vi "dfd_FXP PtByPt Odd Symmetric FIR.vi"(6 "state in":i64[](array[numeric]), 7 "FXPOPs":T5[](array[typedef]) {"source" items=["Coef a/k"=0, "Coef b/v"=7, "Input"=1, "Output"=2, "Multiplicand"=3, "Product"=4, "Sum"=5, "Delay"=6, "Gain"=8]}, 8 "filtering statistics in":T4(array[cluster]) {"statistics information"."min value" format="%.2f"; "statistics information"."max value" format="%.2f"; "Quantizer Source" items=["Coefficients a/k"=0, "Coefficients b/v"=7, "Input"=1, "Output"=2, "Multiplicand"=3, "Product"=4, "Sum"=5, "Delay"=6]}, 10 "coef b (half stored)":i64[](array[numeric]), 11 "x":T7={"value"=0, "wl"=0, "iwl"=0, "Signed"=TRUE} {"value" format="%.0x"}) -> (0 "filtering statistics out":T4(array[cluster]) {"statistics information"."min value" format="%.2f"; "statistics information"."max value" format="%.2f"; "Quantizer Source" items=["Coefficients a/k"=0, "Coefficients b/v"=7, "Input"=1, "Output"=2, "Multiplicand"=3, "Product"=4, "Sum"=5, "Delay"=6]}, 3 "filtered x":T7={"value"=0, "wl"=0, "iwl"=0, "Signed"=TRUE} {"value" format="%.0x"}, 4 "state out":i64[](array[numeric]))   [LabVIEW 2017, in "NI_DigFilter_FXP.lvlib"]
uses:
  <vilib>/addons/Digital Filter Design/NI_DigFilter_FXP.lvlib
  <vilib>/addons/Digital Filter Design/_Objects.llb/dfd_DFXP Data Type (scaler).ctl
  <vilib>/addons/Digital Filter Design/_Objects.llb/dfd_DFXP Operation Parameter.ctl
  <vilib>/addons/Digital Filter Design/_Objects.llb/dfd_Internal Quantization Srcs.ctl
  <vilib>/addons/Digital Filter Design/_Objects.llb/DFD Quantization Sources.ctl
  <vilib>/addons/Digital Filter Design/_Objects.llb/DFD FXP Statistics Data.ctl
  <vilib>/addons/Digital Filter Design/_Objects.llb/dfd_DFXP Data Type (vector).ctl
  <vilib>/addons/Digital Filter Design/NI_DigFilterLicensed.lvlib
panel:
  in  "DFXP type":T1
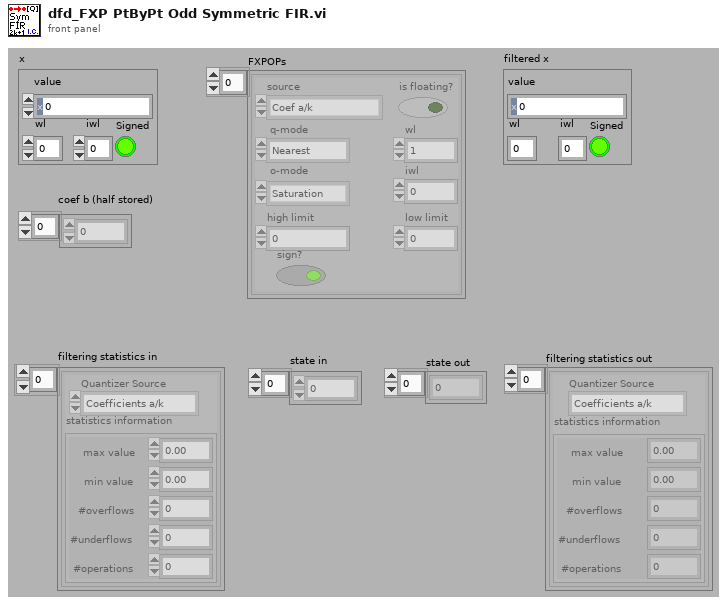
[diagram p1: front panel]
types:
  T1 = typedef "dfd_DFXP Data Type (vector).ctl" = cluster{"Values":i64[], "wl":i16, "iwl":i16}
  T2 = typedef "NI_DigFilterLicensed.lvlib/DFD Quantization Sources.ctl" = u16
  T3 = typedef "NI_DigFilterLicensed.lvlib/DFD FXP Statistics Data.ctl" = cluster{"max value":ext, "min value":ext, "#overflows":i32, "#underflows":i32, "#operations":i32}
  T4 = cluster{"Quantizer Source":T2, "statistics information":T3}[]
  T5 = typedef "dfd_DFXP Operation Parameter.ctl" = cluster{"source":T6, "is floating?":bool, "o-mode":enum16{"Saturation", "Wrap"}, "q-mode":enum16{"Nearest", "Truncation"}, "wl":i16, "high limit":i64, "low limit":i64, "iwl":i16, "sign?":bool}
  T6 = typedef "NI_DigFilterLicensed.lvlib/dfd_Internal Quantization Srcs.ctl" = u16
  T7 = typedef "dfd_DFXP Data Type (scaler).ctl" = cluster{"value":i64, "wl":i16, "iwl":i16, "Signed":bool}
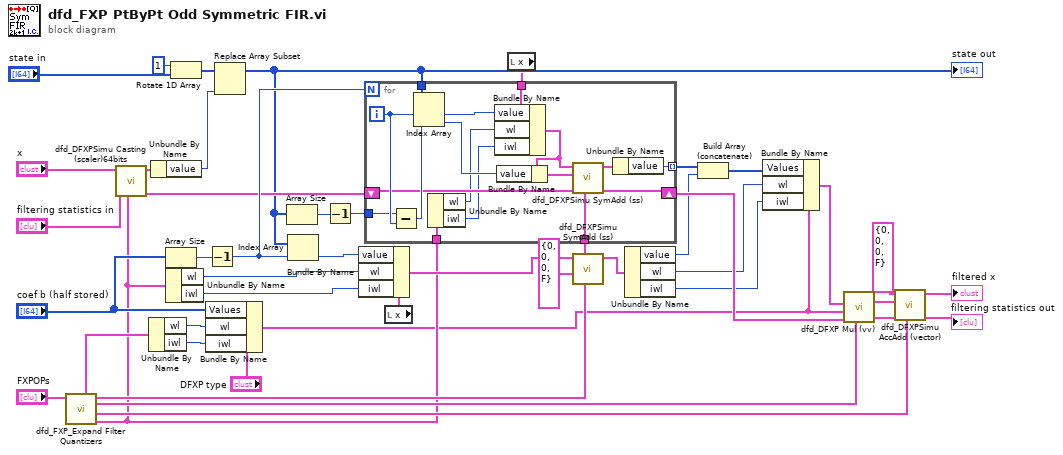
[diagram p0: block diagram]
diagram:
  n1 = call <vilib>:"dfd_FXP_Expand Filter Quantizers.vi"("FXPOPs"="FXPOPs") -> ("Delay"=w8:T5, "Sum"=w32:T5, "Product"=w33:T5, "Multiplicand"=w26:T5, "Coefficient b/v"=w16:T5)  [unwired: 6 out]
  n2 = call <vilib>:"dfd_DFXPSimu Casting (scaler)64bits.vi"("op params"=w8, "filtering statistics in"="filtering statistics in", "Value in"="x") -> ("filtering statistics out"=w29:T4, "Value out"=w20:T7)  [unwired: 1 in, 6 out]
  n3 = Unbundle By Name(w16) -> ("wl"=w13:i16, "iwl"=w12:i16)
  n4 = Unbundle By Name(w20) -> ("value"=w9:i64)
  n5 = Array Size(array="coef b (half stored)") -> (size(s)=w42:i32)
  n6 = Unbundle By Name(w8) -> ("wl"=w11:i16, "iwl"=w10:i16)
  n7 = Rotate 1D Array(1:"state in", 2:1 ("n")) -> (0:w44:i64[])
  n8 = Bundle By Name(cluster="DFXP type", "Values"="coef b (half stored)", "wl"=w13, "iwl"=w12) -> (w5:T1)
  n9 = Decrement(x=w42) -> (x-1=w31:i32)
  n10 = Replace Array Subset(array=w44, new element=w9) -> (w22:i64[])  [unwired: 1 in]
  "state out" <- w22
  n11 = Array Size(array=w22) -> (size(s)=w40:i32)
  n12 = Index Array(array=w22, index=w31) -> (element=w27:i64)
  n13 = Decrement(x=w40) -> (x-1=w38:i32)
  n14 = local read "x"() -> (w14:T7)
  n15 = Bundle By Name(cluster=w14, "value"=w27, "wl"=w11, "iwl"=w10) -> (w15:T7)
  n16 = local read "x"() -> (w7:T7)
  n17 = for {
    N: w31 -> [_]
    tunnel: w22 -> [w61]
    tunnel: w38 -> [w58]
    tunnel: [w45] -> w24 mode=indexing
    shift-right: [w56] -> w28
    shift-left: w29 -> [w57]
    tunnel: w26 -> [w55]
    tunnel: w8 -> [w51]
    tunnel: w7 -> [w47]
    i -> [w60]
    n18 = Subtract(x=w58, y=w60) -> (x-y=w59:i32)
    n19 = Index Array(array=w61, index #1=w60, index #2=w59) -> (element #1=w54:i64, element #2=w53:i64)
    n20 = Unbundle By Name(w51) -> ("wl"=w50:i16, "iwl"=w49:i16)
    n21 = Bundle By Name(cluster=w47, "value"=w54, "wl"=w50, "iwl"=w49) -> (w46:T7)
    n22 = Bundle By Name(cluster=w46, "value"=w53) -> (w48:T7)
    n23 = call <vilib>:"dfd_DFXPSimu SymAdd (ss).vi"("op params"=w55, "filtering statistics in"=w57, "value in 2"=w48, "value in 1"=w46) -> ("filtering statistics out"=w56:T4, "value out"=w52:T7)  [unwired: 2 in, 4 out]
    n24 = Unbundle By Name(w52) -> ("value"=w45:i64)
  }
  n25 = call <vilib>:"dfd_DFXPSimu SymAdd (ss).vi"("op params"=w26, "value in 2"=T7 {"value"=0, "wl"=0, "iwl"=0, "Signed"=FALSE} ("value2 in"), "value in 1"=w15) -> ("value out"=w18:T7)  [unwired: 2 in, 6 out]
  n26 = Unbundle By Name(w18) -> ("value"=w6:i64, "wl"=w3:i16, "iwl"=w2:i16)
  n27 = Build Array (concatenate)(w24, w6) -> (w4:i64[])
  n28 = Bundle By Name(cluster=w5, "Values"=w4, "wl"=w3, "iwl"=w2) -> (w1:T1)
  n29 = call <vilib>:"dfd_DFXP Mul (vv).vi"("op params"=w33, "filtering statistics in"=w28, "Value in 2"=w5, "Value in"=w1) -> ("filtering statistics out"=w34:T4, "Value out"=w35:T1)  [unwired: 6 out]
  n30 = call <vilib>:"dfd_DFXPSimu AccAdd (vector).vi"("op params"=w32, "filtering statistics in"=w34, "addends"=w35, "acc in"=T7 {"value"=0, "wl"=0, "iwl"=0, "Signed"=FALSE}) -> ("filtering statistics out"=→"filtering statistics out":T4, "acc out"=→"filtered x":T7)  [unwired: 1 in, 5 out]
